vi "SRV_TCP Write Data.vi"(8 "error in":errorcluster, 9 "timeout ms (100)":i32=100, 10 "data in":string, 11 "connection ID":refnum<k5>) -> (0 "error out":errorcluster, 2 "bytes written":i32, 3 "connection ID out":refnum<k5>)   [LabVIEW 2009]
doc: "Writes data to a TCP network connection."
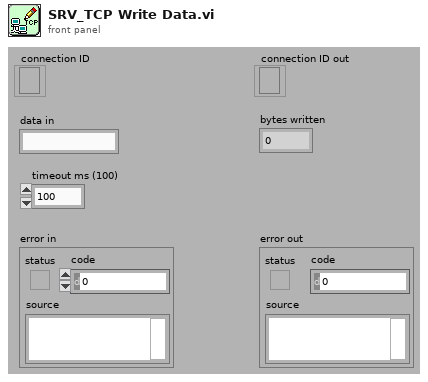
[diagram p1: front panel]
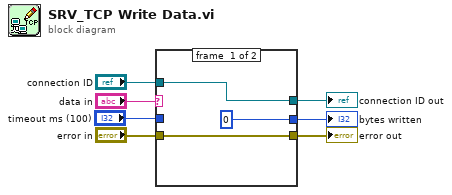
[diagram p0: block diagram]
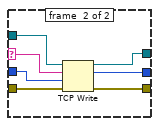
[diagram p2: hidden frame]
diagram:
  n1 = case shown="Default" "data in" {
    selector: "data in" -> [_ w12]
    tunnel: [w10 w13] -> w7
    tunnel: [w9 w17] -> w6
    tunnel: "error in" -> [w9 w16]
    tunnel: "connection ID" -> [w10 w14]
    tunnel: [0 ("bytes written") w15] -> w3
    tunnel: "timeout ms (100)" -> [_ w11]
    frame #0 {
    }
    frame #1 {
      n2 = TCP Write(connection ID=w14, data in=w12, error in (no error)=w16, 9:w11) -> (connection ID out=w13:refnum<k5>, bytes written=w15:i32, error out=w17:errorcluster)
    }
  }
  "connection ID out" <- w7
  "error out" <- w6
  "bytes written" <- w3
